vi "viewer.vi"() -> ()   [LabVIEW 2013]
uses:
  ExperimentVariables/Variable_Status.ctl
  DDS drivers v3/DDS RAM mode.ctl
  <vilib>/ni845x/ni845x.llb/ni845xControl.ctl
  DDS drivers v3/DDS box device reference.ctl
  DDS drivers v3/DDS Settings.ctl
  DDS drivers v3/DDS Profile Settings.ctl
  ExperimentVariables/current_variables_table.ctl
panel:
  out "Background Array":u16[][](array[numeric])
  in  "Tab Control":T1(tab)=enum."Filters"
  in  "Experiment data directory":path
  in  "Measurement":dbl
  in  "Cycle":dbl
  in  "Select which iteration to view via variables: name, value":cluster{"Name":string, "Enum":enum16{""}}[](array[cluster])
  out "Variable Status":T2={"Variables (Indicator)"=[["x", "0.000", "0", "145.000"], ["y", "0.000", "0", "0.001"], ["z", "0.000", "0", "0.000"]], "Total Iterations"=0, "Current Iteration"=0, "Current measurement"=0, "wait loops"=0}
  out "HSDIO Status":T4={"Channel List"="0,1,3,4,5", "Loaded Waveforms"=["Hex_Array_Loading"], "A waveform was padded"=FALSE, "final script this iteration"="script script1\r\nGenerate w00000000\r\nWait 311999\nGenerate w00000008\r\nWait 87999\nGenerate w0000001A\r\nWait 11999\nGenerate w00000019\r\nWait 99999\nGenerate w00000011\r\nWait 99999\nGenerate w00000012\r\nWait 399999\nGenerate w00000031\r\nWait 199999\nGenerate w00000011\r\nWait 1799999\nGenerate w00000010\r\nWait 1387999\nGenerate w00000000\r\nWait 35599998\nGenerate w00000000\r\nGenerate w00000000\r\nend script\r\n"}
  out "DDS Initialized":bool=TRUE
  in  "DDS Box Select Tabs":enum32{"DDS Box 1", "DDS Box 2"}(tab)
  in  "DDS Settings Box 1":T5={"DDS Profile Settings"=[], "RAM Enable"=[], "RAM Default Profile"=[], "DDS box device reference"={"NI USB-8451 device reference"="", "DIO port"=0, "Serial Clock Rate [kHz]"=1000, "Channels Settings"=[{"Ref Clock Rate [MHz]"=1000.0, "Full Scale Output Power [dBm]"=0.0}, {"Ref Clock Rate [MHz]"=1000.0, "Full Scale Output Power [dBm]"=0.0}, {"Ref Clock Rate [MHz]"=1000.0, "Full Scale Output Power [dBm]"=0.0}, {"Ref Clock Rate [MHz]"=1000.0, "Full Scale Output Power [dBm]"=0.0}]}, "RAM Destination"=[], "DDS Power"=[FALSE, FALSE, FALSE, FALSE]}
  in  "DDS Settings Box 2":T5={"DDS Profile Settings"=[], "RAM Enable"=[], "RAM Default Profile"=[], "DDS box device reference"={"NI USB-8451 device reference"="", "DIO port"=0, "Serial Clock Rate [kHz]"=1000, "Channels Settings"=[{"Ref Clock Rate [MHz]"=1000.0, "Full Scale Output Power [dBm]"=0.0}, {"Ref Clock Rate [MHz]"=1000.0, "Full Scale Output Power [dBm]"=0.0}, {"Ref Clock Rate [MHz]"=1000.0, "Full Scale Output Power [dBm]"=0.0}, {"Ref Clock Rate [MHz]"=1000.0, "Full Scale Output Power [dBm]"=0.0}]}, "RAM Destination"=[], "DDS Power"=[FALSE, FALSE, FALSE, FALSE]}
  in  "Image Display Maximum":u16 caption="Display Maximum"
  in  "Image Display Minimum":u16 caption="Display Minimum"
  in  "Image Dynamic scaling":bool caption="Dynamic scaling"
  out "Set?":bool
  in  "Set Current Average Image as Background":bool
  out "Image Array for whole experiment":T10[][][][](array[plugin-control]) caption="(Cycles, Iterations, Measurements, Shots, scaling above)"
  out "Average of All Images from experiment":T10(plugin-control) caption="Average of All Images (dynamically scaled)"
  in  "Image Background":dbl
  out "ROI Pixel Count":u64[][][][](array[numeric])
  out "Histogram of ROI Sum over All Images":T11(graph)
  in  "# intervals (mutli-shot)":i32=128
  out "Camera Temperature":dbl format="%_5g"
  out "Image Array for most recent measurement":T10[](array[plugin-control]) caption="(by shot, dynamically scaled)"
  in  "Background image Dynamic scaling":bool caption="Dynamic scaling"
  in  "Background Image Display Maximum":u16 caption="Display Maximum"
  in  "Background Image Display Minimum":u16 caption="Display Minimum"
  out "Backgound Subtracted Average Image":T10(plugin-control) caption="(dynamic scaling)"
  out "Background Subtracted Image Array":T10[][][][](array[plugin-control]) caption="(Cycles, Iterations, Measurements, Shots, scaling above)"
  in  "Run Background Subtraction":bool
  out "Background Image":T10(plugin-control) caption="(dynamic scaling)"
  out "Counters Chart":u32[][](graph)
  out "current counter totals":u32[](array[numeric])
  in  "Notes Cluster":cluster{"Notes":string[][], "Comments":string}
  out "Experiment is Running":bool
  out "Error LED":bool caption="Error"
  # "Ch. 1"
  # "Ch. 2"
  # "Ch. 3"
  # "Ch. 4"
  # "Ch. 1"
  # "Ch. 2"
  # "Ch. 3"
  # "Ch. 4"
  # "Static Arrays"
  # "Ch. 1"
  # "Ch. 2"
  # "Ch. 3"
  # "Ch. 4"
  # "Ch. 1"
  # "Ch. 2"
  # "Ch. 3"
  # "Ch. 4"
  # "Ch. 1"
  # "Ch. 2"
  # "Ch. 3"
  # "Ch. 4"
  # "Static Arrays"
  # "Ch. 1"
  # "Ch. 2"
  # "Ch. 3"
  # "Ch. 4"
  # "Notes will be auto-evaluated and will be saved with comments in each experiment directory."
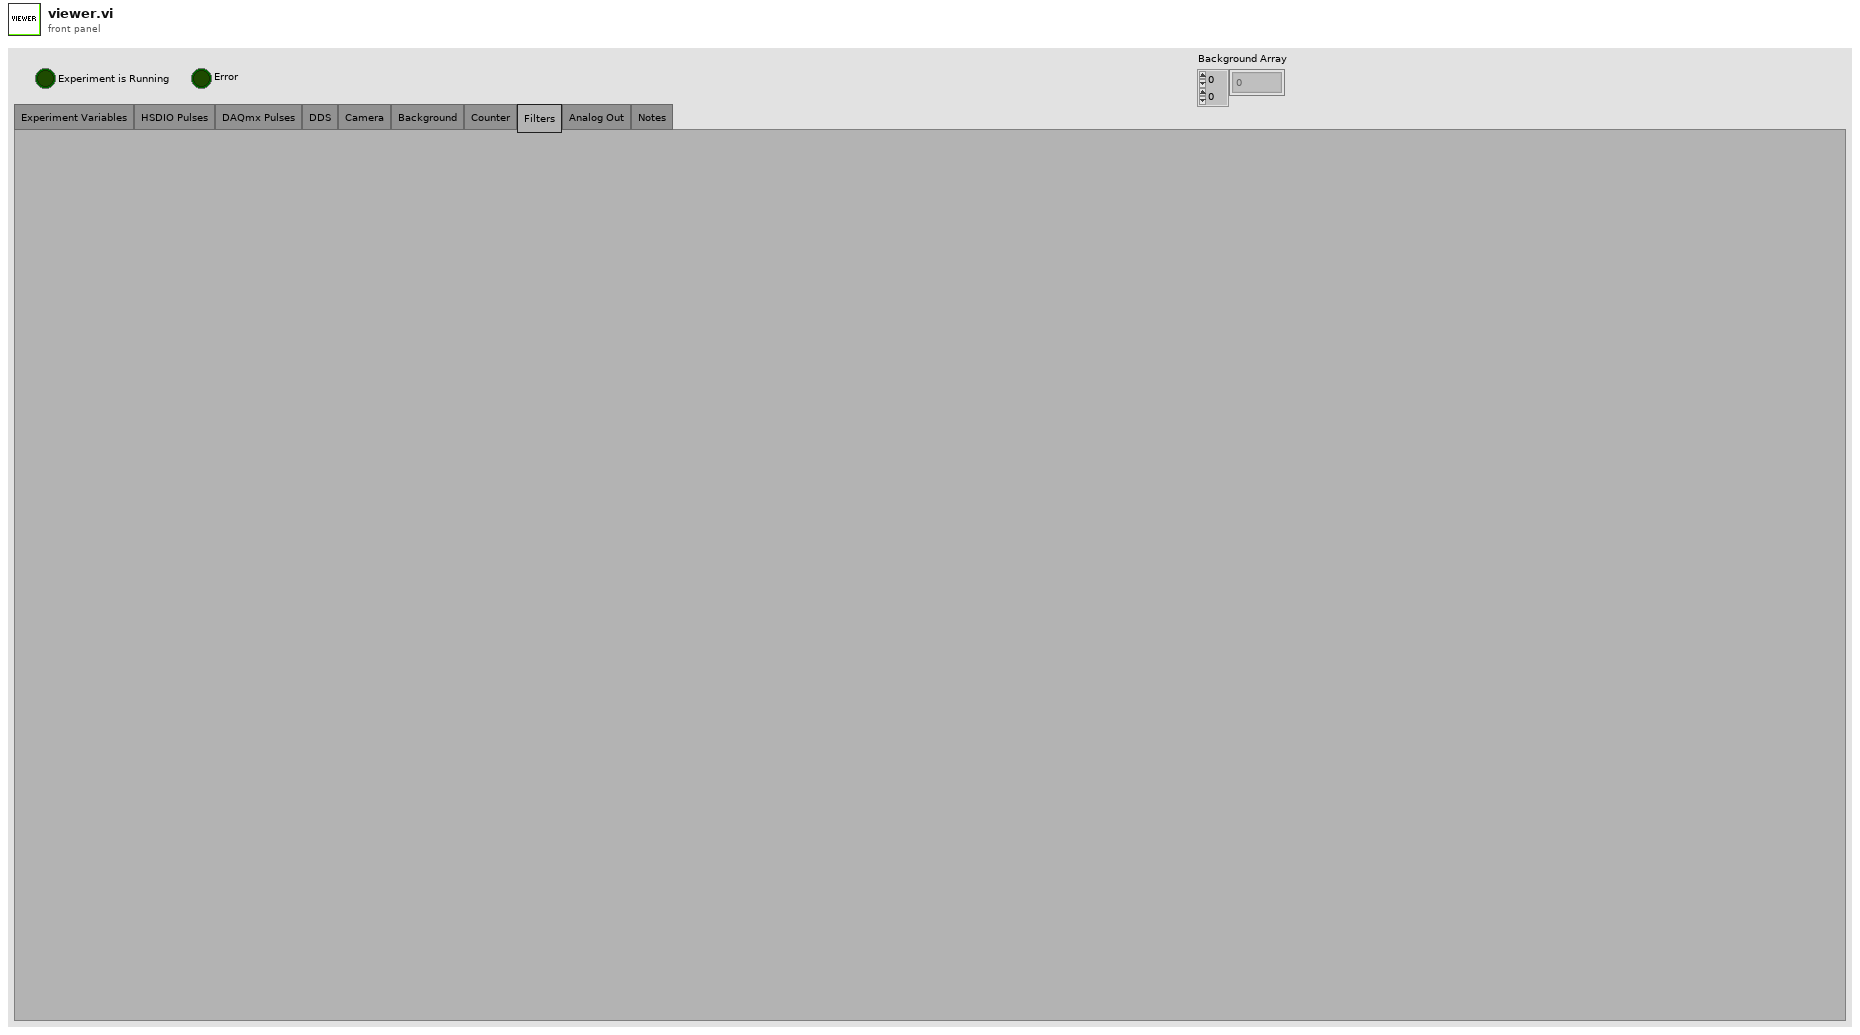
[diagram p1: front panel]
types:
  T1 = enum32{"Experiment Variables", "HSDIO Pulses", "DAQmx Pulses", "DDS", "Camera", "Background", "Counter", "Filters", "Analog Out", "Notes"}
  T2 = typedef "ExperimentVariables.lvclass/Variable_Status.ctl" = cluster{"Variables (Indicator)":T3, "Total Iterations":u32, "Current Iteration":u32, "Current measurement":u32, "wait loops":u32}
  T3 = typedef "ExperimentVariables.lvclass/current_variables_table.ctl" = string[][]
  T4 = cluster{"Channel List":string, "Loaded Waveforms":string[], "A waveform was padded":bool, "final script this iteration":string}
  T5 = typedef "DDS Settings.ctl" = cluster{"DDS Profile Settings":T6[], "RAM Enable":bool[], "RAM Default Profile":cluster{"Frequency [MHz]":string, "Amplitude [dBm]":string, "Phase Offset [rad]":string}[], "DDS box device reference":T8, "RAM Destination":u8[], "DDS Power":bool[]}
  T6 = typedef "DDS Profile Settings.ctl" = cluster{"RAM Mode":T7[], "Zero-crossing":bool[], "No Dwell High":bool[], "RAM Static Array Ch. 1":dbl[], "Function/Static":bool[], "Single Tone Profiles":cluster{"Frequency [MHz]":string, "Amplitude [dBm]":string, "Phase Offset [rad]":string}[], "RAM Function Settings":string[][], "RAM Static Array Ch. 2":dbl[], "RAM Static Array Ch. 3":dbl[], "RAM Static Array Ch. 4":dbl[]}
  T7 = typedef "DDS RAM mode.ctl" = enum16{"Direct Switch", "Ramp Up", "Bidirectional Ramp", "Continuous Bidirectional Ramp", "Continuous Recirculate", "Direct Switch 2", "Direct Switch 3", "Direct Switch 4"}
  T8 = typedef "DDS box device reference.ctl" = cluster{"NI USB-8451 device reference":T9, "DIO port":u8, "Serial Clock Rate [kHz]":u16, "Channels Settings":cluster{"Ref Clock Rate [MHz]":dbl, "Full Scale Output Power [dBm]":dbl}[]}
  T9 = typedef "ni845xControl.ctl" = refnum<k21>
  T10 = typedef "IMAQ Image.ctl" = refnum<image>
  T11 = cluster{"X Values":dbl[], "Histogram: h(x)":i32[]}
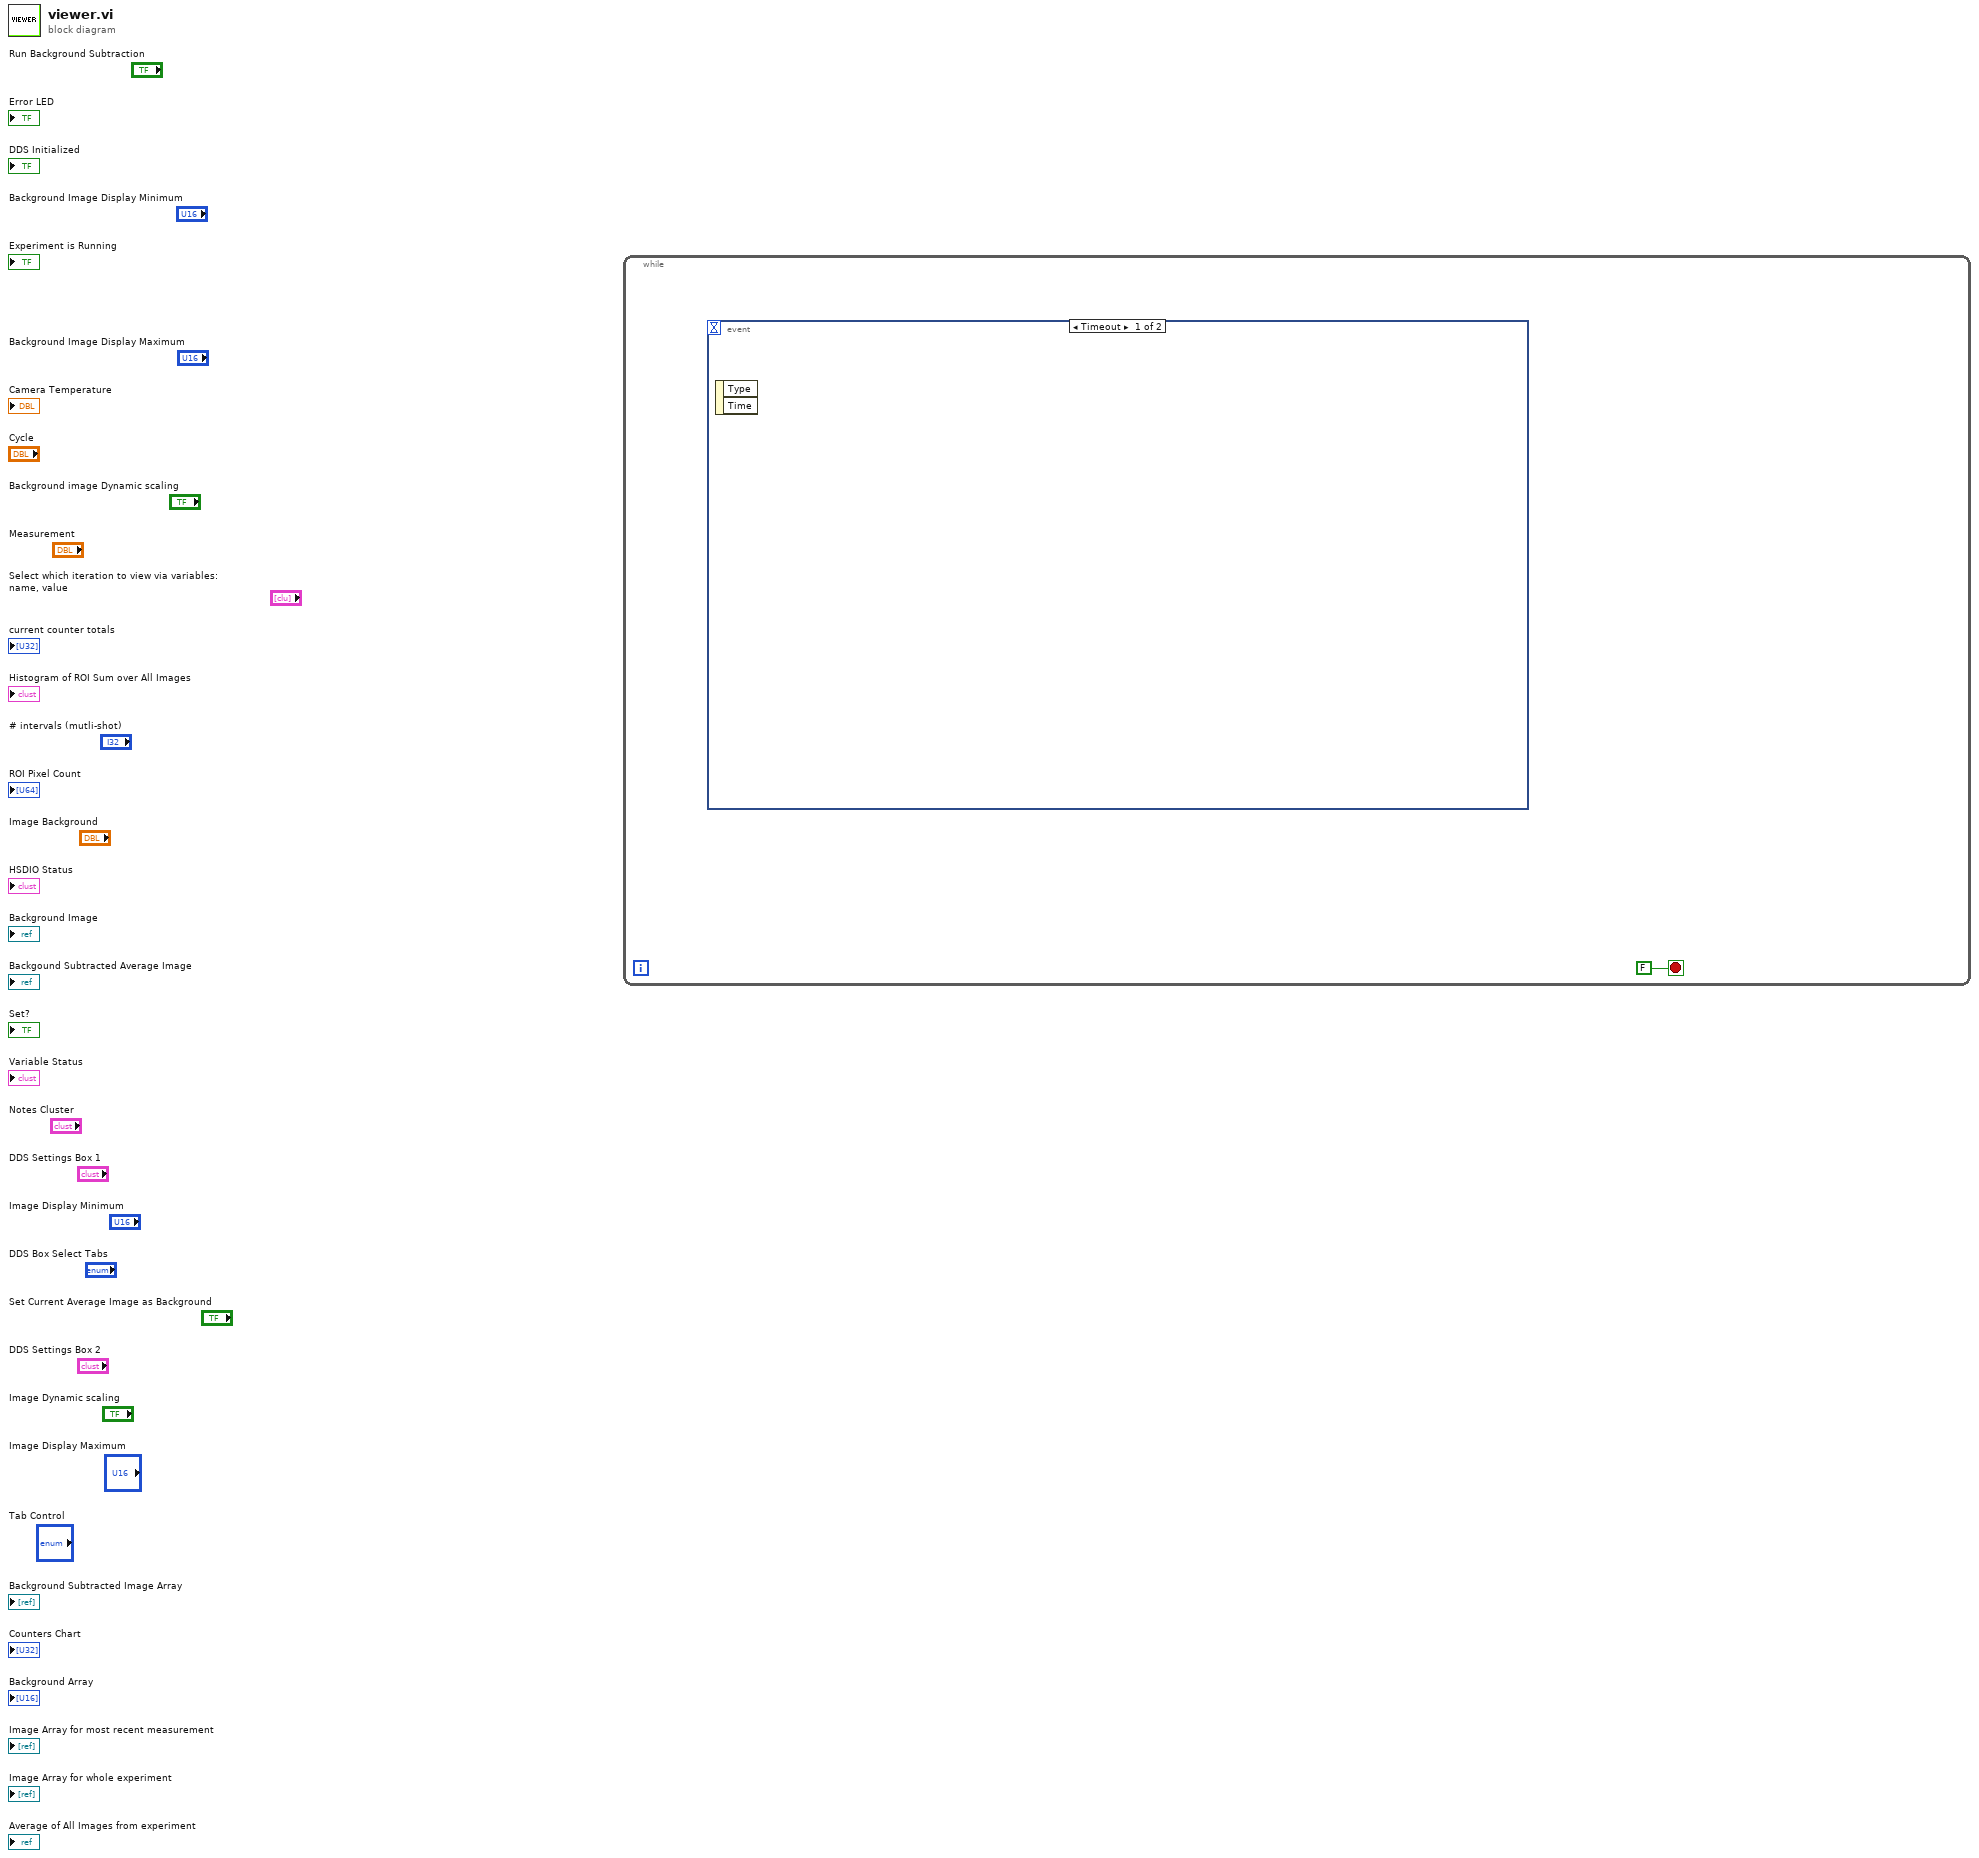
[diagram p0: block diagram]
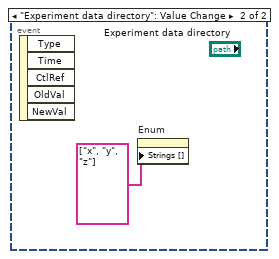
[diagram p2: hidden frame]
diagram:
  n1 = while {
    stop <- FALSE stop-if-true
    n2 = event shown="[0] Timeout" {
      selector: _ -> [_ _]
      dyn-events: _ -> [_ _]
      timeout: _ -> [_ _]
      event Timeout {
        n3 = event-data() -> ()  [unwired: 1 in, 2 out]
      }
      event "Experiment data directory": Value Change {
        n4 = event-data() -> ()  [unwired: 1 in, 5 out]
        n5 = property on="Enum" class="Enum (strict)"("Strings []"=string[] ["x", "y", "z"]) -> ()  [unwired: 2 in, 2 out]
      }
    }
  }
